vi "put_tablecloth.vi"(8 "error in (no error)":errorcluster, 11 "Table in":refnum<class "Table.lvclass">) -> (0 "error out":errorcluster, 2 "result":string, 3 "Table out":refnum<class "Table.lvclass">)   [LabVIEW 2021, in "Table.lvclass"]
uses:
  Table.lvclass
  Table.lvclass/Table.ctl
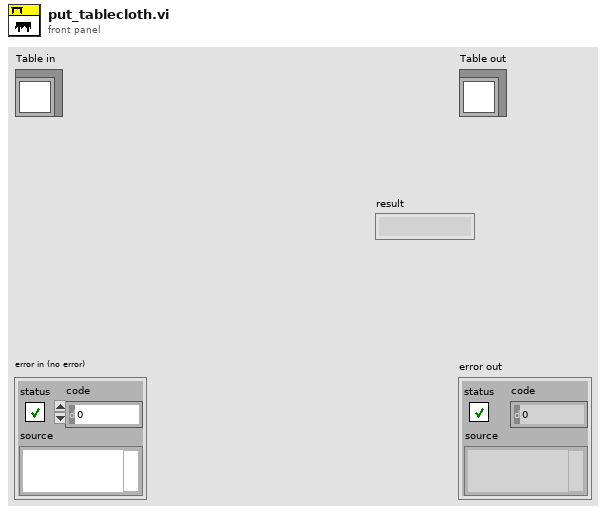
[diagram p1: front panel]
types:
  T1 = typedef "Table.lvclass/TableclothType.ctl" = u16
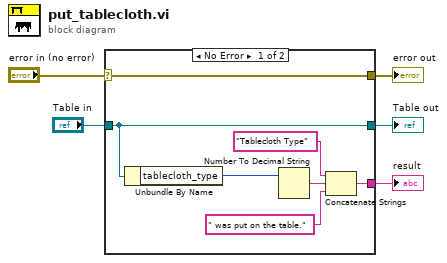
[diagram p0: block diagram]
diagram:
  n1 = case shown="No Error" "error in (no error)" {
    selector: "error in (no error)" -> [w12 w14]
    tunnel: [w12 w14] -> w4
    tunnel: [w8 w13] -> w2
    tunnel: "Table in" -> [w8 w13]
    tunnel: [w6 _] -> w1
    frame No Error {
      n2 = Unbundle By Name(w8) -> ("tablecloth_type"=w9:T1)
      n3 = Number To Decimal String(number=w9) -> (decimal integer string=w10:string)  [unwired: 1 in]
      n4 = Concatenate Strings("Tablecloth Type", w10, " was put on the table.") -> (w6:string)
    }
    frame Error {
    }
  }
  "error out" <- w4
  "Table out" <- w2
  "result" <- w1
